vi "TTA_EXA_Single_Sweep.vi"(0 "VISA resource In":refnum<visa-resource-name>, 11 "error in":errorcluster) -> (4 "VISA resource Out":refnum<visa-resource-name>, 6 "OPC?":bool, 15 "error out":errorcluster)   [LabVIEW 2016]
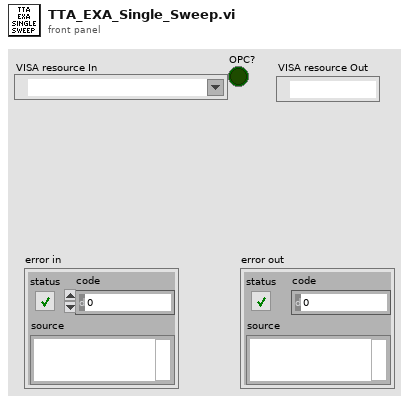
[diagram p1: front panel]
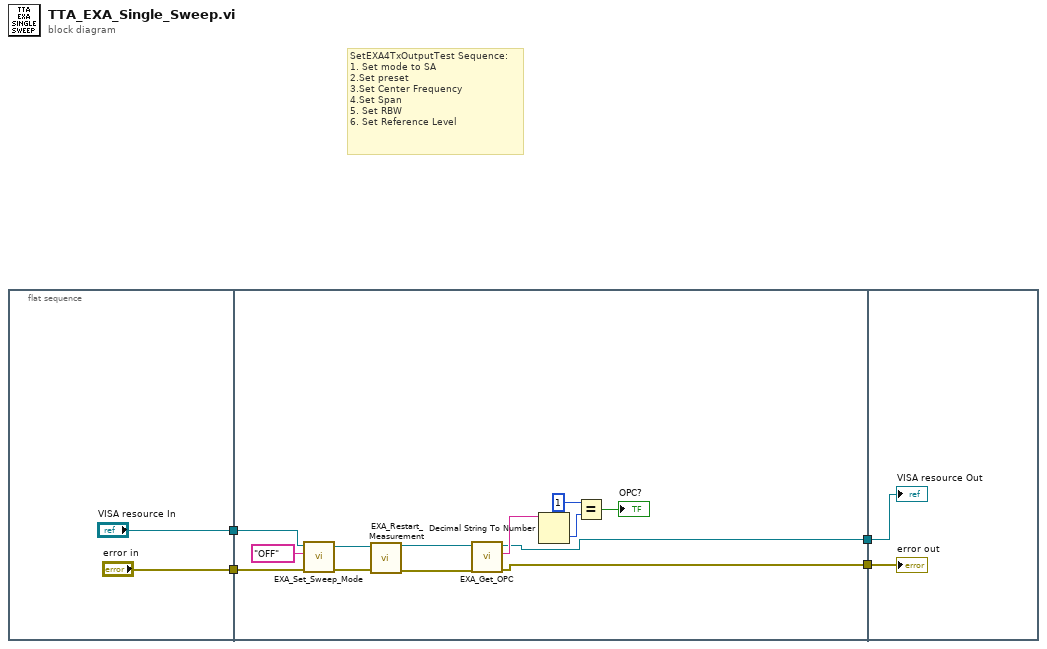
[diagram p0: block diagram]
diagram:
  # "SetEXA4TxOutputTest Sequence:\n1. Set mode to SA\n2.Set preset\n3.Set Center Frequency\n4.Set Span\n5. Set RBW\n6. Set Reference Level"
  n1 = flat-sequence {
    tunnel: ["error in"] -> w4
    tunnel: ["VISA resource In"] -> w3
    tunnel: w4 -> [w19]
    tunnel: w3 -> [w18]
    tunnel: [w8] -> w2
    tunnel: [w7] -> w1
    tunnel: w2 -> [w21]
    tunnel: w1 -> [w20]
    frame #0 {
    }
    frame #1 {
      n2 = call "EXA_Set_Sweep_Mode.vi"("error in"=w19, "Continous"="OFF", "VISA resource name"=w18) -> ("error out"=w16:errorcluster, "VISA resource name"=w13:refnum<visa-resource-name>)  [unwired: 7 in]
      n3 = call "EXA_Restart_Measurement.vi"("error in"=w16, "VISA resource name"=w13) -> ("error out"=w15:errorcluster, "VISA resource name"=w14:refnum<visa-resource-name>)  [unwired: 8 in]
      n4 = call "EXA_Get_OPC.vi"("error in"=w15, "VISA resource name"=w14) -> ("error out"=w7:errorcluster, "read buffer"=w12:string, "VISA resource name"=w8:refnum<visa-resource-name>)  [unwired: 7 in]
      n5 = Decimal String To Number(string=w12) -> (number=w11:i32)  [unwired: 2 in, 1 out]
      n6 = Equal?(x=1, y=w11) -> (x = y?=→"OPC?":bool)
    }
    frame #2 {
      "VISA resource Out" <- w21
      "error out" <- w20
    }
  }
